vi "write bit file.vi"() -> (3 "Success":bool)   [LabVIEW 2018]
uses:
  Dll1_x64_191014_0/Dll1_x64_191014_0.lvlib
panel:
  out "progress":dbl(slide) scale=0.0..100.0
  out "status":string
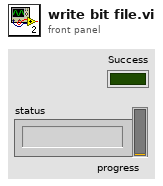
[diagram p1: front panel]
types:
  T1 = enum32{"invalid app kind", "Development System", "Run Time System", "Student Edition", "Embedded LabVIEW", "Evaluation", "Custom"}
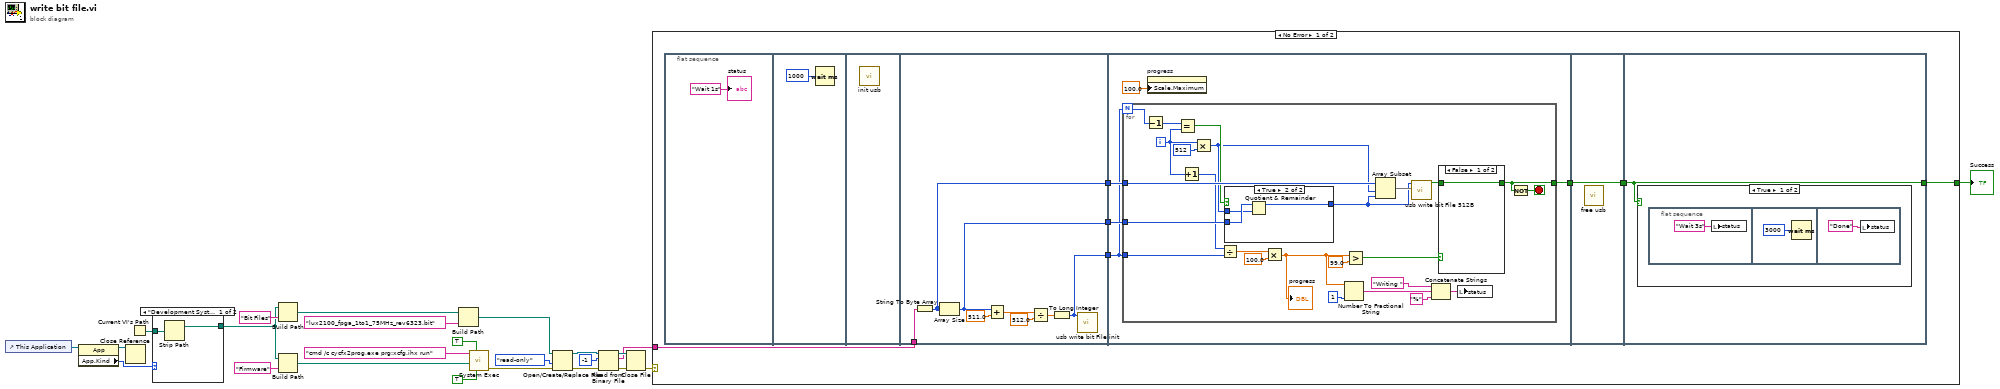
[diagram p0: block diagram]
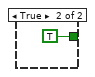
[diagram p2: hidden frame]
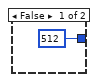
[diagram p3: hidden frame]
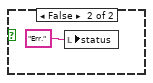
[diagram p4: hidden frame]
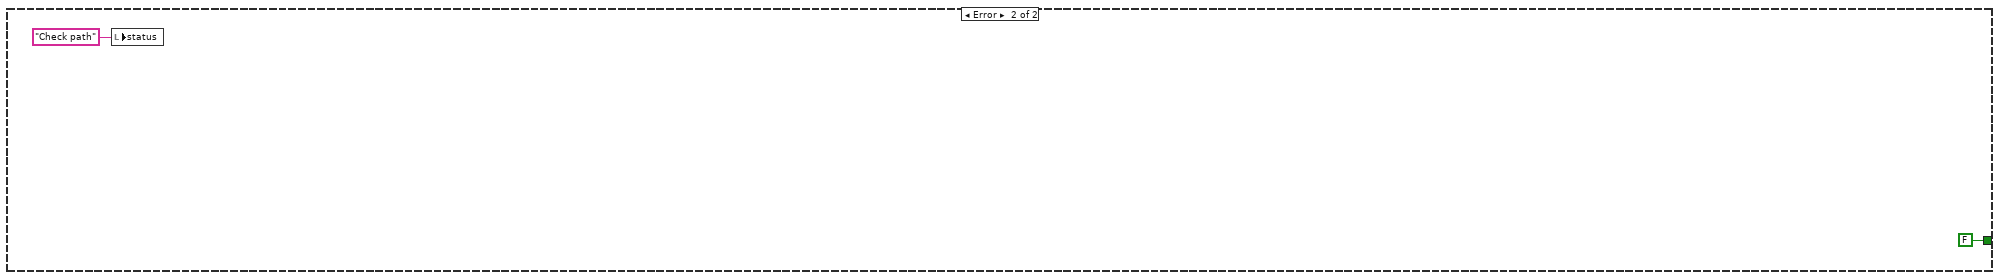
[diagram p5: hidden frame]
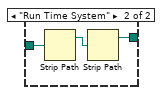
[diagram p6: hidden frame]
diagram:
  n1 = control-ref of="This Application"() -> (w21:refnum<vi>)
  n2 = property class="App"(reference=w21) -> (reference out=w22:refnum<vi>, "App.Kind"=w23:T1)  [unwired: 1 in, 1 out]
  n3 = Close Reference(reference=w22) -> ()  [unwired: 1 in, 1 out]
  n4 = Current VI's Path() -> (path=w24:path)
  n5 = case shown="\"Development System\", Default" w23 {
    tunnel: w24 -> [w26 w29]
    tunnel: [w25 w27] -> w5
    frame "Development System", Default {
      n6 = Strip Path(path=w26) -> (stripped path=w25:path)  [unwired: 1 out]
    }
    frame "Run Time System" {
      n7 = Strip Path(path=w29) -> (stripped path=w28:path)  [unwired: 1 out]
      n8 = Strip Path(path=w28) -> (stripped path=w27:path)  [unwired: 1 out]
    }
  }
  n9 = Build Path(base path=w5, name or relative path="Bit Files") -> (appended path=w11:path)
  n10 = Build Path(base path=w5, name or relative path="Firmware") -> (appended path=w20:path)
  n11 = Build Path(base path=w11, name or relative path="lux2100_fpga_1to1_75MHz_rev6323.bit") -> (appended path=w10:path)
  n12 = call <vilib>:"System Exec.vi"("run minimized? (F)"=TRUE, "wait until completion? (T)"=TRUE, "working directory"=w20, "command line"="cmd /c cycfx2prog.exe prg:xcfg.ihx run") -> ("error out"=w2:errorcluster)  [unwired: 4 in, 3 out]
  n13 = Open/Create/Replace File(file path (use dialog)=w10, error in=w2, access (0:read/write)=enum16{"read/write", "read-only", "write-only"}."read-only") -> (refnum out=w15:refnum<file>, error out=w13:errorcluster)  [unwired: 3 in, 1 out]
  n14 = Read from Binary File(8:w13, 10:-1 ("count (1)"), 11:w15) -> (0:w12:errorcluster, 2:w4:string, 3:w14:refnum<file>)  [unwired: 3 in, 1 out]
  n15 = Close File(refnum=w14, error in=w12) -> (error out=w1:errorcluster)  [unwired: 1 out]
  n16 = case shown="No Error" w1 {
    tunnel: w4 -> [w31 _]
    tunnel: [w30 FALSE ("function return")] -> w3
    frame No Error {
      n17 = flat-sequence {
        tunnel: [w42] -> w36
        tunnel: [w41] -> w35
        tunnel: [w40] -> w34
        tunnel: w31 -> [w39]
        tunnel: w36 -> [w49]
        tunnel: w35 -> [w51]
        tunnel: w34 -> [w50]
        tunnel: [w47] -> w33
        tunnel: [w83] -> w32
        tunnel: w33 -> [w83]
        tunnel: w32 -> [w84]
        tunnel: [w84] -> w30
        frame #0 {
          "status" <- "Wait 1s" ("status")
        }
        frame #1 {
          n18 = Wait (ms)(milliseconds to wait=u32 1000) -> ()  [unwired: 1 out]
        }
        frame #2 {
          n19 = call "init usb.vi"() -> ()  [unwired: 12 in]
        }
        frame #3 {
          n20 = String To Byte Array(string=w39) -> (unsigned byte array=w40:u8[])
          n21 = Array Size(array=w40) -> (size(s)=w41:i32)
          n22 = Add(x=w41, y=511.0) -> (x+y=w45:dbl)
          n23 = Divide(x=w45, y=512.0) -> (x/y=w46:dbl)
          n24 = To Long Integer(number=w46) -> (32bit integer=w42:i32)
          n25 = call "usb write bit File init.vi"("blkCnt_512B"=w42) -> ()  [unwired: 11 in]
        }
        frame #4 {
          n26 = for {
            N: w49 -> [w73]
            tunnel: w50 -> [w76]
            tunnel: w51 -> [w70]
            tunnel: w49 -> [w65]
            tunnel: [w52] -> w47
            i -> [w67]
            stop <- w53 stop-if-true
            n27 = Decrement(x=w73) -> (x-1=w72:i32)
            n28 = Equal?(x=w72, y=w67) -> (x = y?=w71:bool)
            n29 = Increment(x=w67) -> (x+1=w66:i32)
            n30 = Multiply(x=w67, y=512) -> (x*y=w69:i32)
            n31 = Divide(x=w66, y=w65) -> (x/y=w59:dbl)
            n32 = case shown="True" w71 {
              tunnel: [512 ("len") w80] -> w68
              tunnel: w70 -> [_ w82]
              tunnel: w69 -> [_ w81]
              frame False {
              }
              frame True {
                n33 = Quotient & Remainder(x=w82, y=w81) -> (x-y*floor(x/y)=w80:i32)  [unwired: 1 out]
              }
            }
            n34 = Multiply(x=w59, y=100.0) -> (x*y=w57:dbl)
            "progress" <- w57
            n35 = Number To Fractional String(number=w57, precision (6)=i16 1) -> (F-format string=w62:string)  [unwired: 2 in]
            n36 = Greater?(x=w57, y=99.0) -> (0:w55:bool)
            n37 = Array Subset(array=w76, index=w69, length=w68) -> (w74:u8[])
            n38 = call "usb write bit File 512B.vi"("bin"=w74, "len"=w68) -> ("function return"=w54:bool)  [unwired: 8 in, 1 out]
            n39 = Concatenate Strings("Writing " ("status"), w62, "%" ("string")) -> (w60:string)
            n40 = case shown="False" w55 {
              tunnel: w54 -> [w77 _]
              tunnel: [w77 TRUE ("function return")] -> w52
              frame False {
              }
              frame True {
              }
            }
            n41 = local write "status"(w60) -> ()
            n42 = Not(x=w52) -> (.not. x?=w53:bool)
          }
          n43 = property on="progress" class="Slide (strict)"("Scale.Maximum"=100.0 ("Scale.Range:Maximum")) -> ()  [unwired: 2 in, 2 out]
        }
        frame #5 {
          n44 = call "free usb.vi"() -> ()  [unwired: 12 in]
        }
        frame #6 {
          n45 = case shown="True" w84 {
            frame True {
              n46 = flat-sequence {
                frame #0 {
                  n47 = local write "status"("Wait 3s" ("status")) -> ()
                }
                frame #1 {
                  n48 = Wait (ms)(milliseconds to wait=u32 3000) -> ()  [unwired: 1 out]
                }
                frame #2 {
                  n49 = local write "status"("Done" ("status")) -> ()
                }
              }
            }
            frame False {
              n50 = local write "status"("Err." ("status")) -> ()
            }
          }
        }
      }
    }
    frame Error {
      n51 = local write "status"("Check path" ("status")) -> ()
    }
  }
  "Success" <- w3
